vi "Create a constant from variant.vi"(5 "Terminal Sink":refnum<vi>, 6 "relative position/next to refnum":T1, 8 "error in (no error)":errorcluster, 10 "Constant Data":variant, 11 "Diagram":refnum<vi>) -> (0 "error out":errorcluster, 2 "Terminal":refnum<vi>, 3 "Const Refnum":refnum<vi>)   [LabVIEW 2018, in "Scripting Tools.lvlib"]
doc: "Create a constant on the block diagram with name and type of <b>Constant Data</b>."
uses:
  Scripting Tools.lvlib
  <vilib>/Utility/miscctls.llb/LVPointTypeDef.ctl
  <vilib>/Utility/VariantDataType/VariantType.lvlib
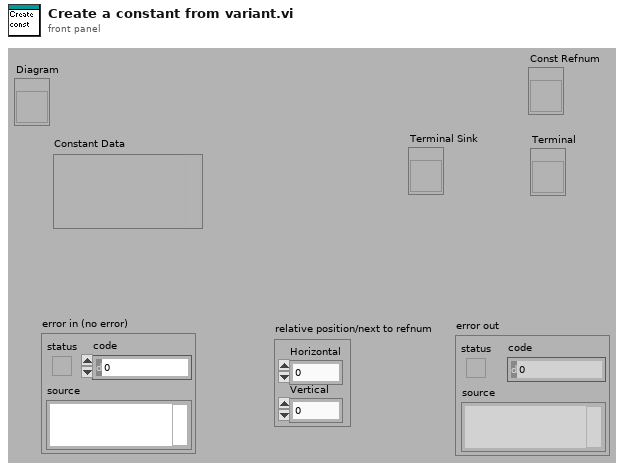
[diagram p1: front panel]
types:
  T1 = typedef "LVPointTypeDef.ctl" = cluster{"Horizontal":i16, "Vertical":i16}
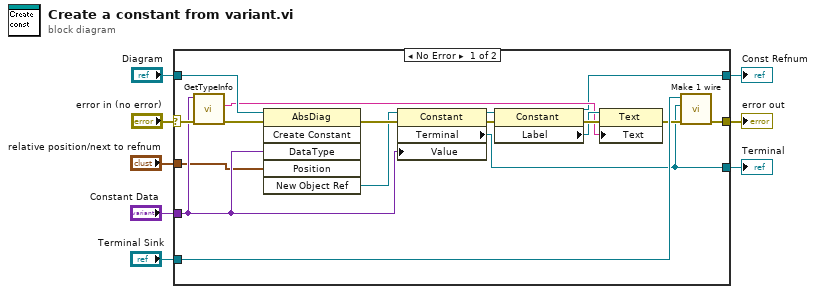
[diagram p0: block diagram]
diagram:
  n1 = case shown="No Error" "error in (no error)" {
    selector: "error in (no error)" -> [w17 w26]
    tunnel: [w25 w26] -> w7
    tunnel: "Constant Data" -> [w15 _]
    tunnel: "relative position/next to refnum" -> [w11 _]
    tunnel: "Terminal Sink" -> [w24 _]
    tunnel: "Diagram" -> [w23 _]
    tunnel: [w9 _] -> w2
    tunnel: [w12 _] -> w1
    frame No Error {
      n2 = call <vilib>:"GetTypeInfo.vi"("error in (no error)"=w17, "Variant"=w15) -> ("error out"=w16:errorcluster, "Name"=w14:string)  [unwired: 8 out]
      n3 = invoke class="AbsDiag" method="Create Constant"(reference=w23, error in=w16, "DataType"=w15, "Position"=w11) -> (error out=w22:errorcluster, "New Object Ref"=w21:refnum<vi>)  [unwired: 2 in, 4 out]
      n4 = property class="Constant"(reference=w21, error in=w22, "Value"=w15) -> (reference out=w20:refnum<vi>, error out=w10:errorcluster, "Terminal"=w9:refnum<vi>)
      n5 = property class="Constant"(reference=w20, error in=w10) -> (reference out=w12:refnum<vi>, error out=w19:errorcluster, "Label"=w18:refnum<vi>)
      n6 = property class="Text"(reference=w18, error in=w19, "Text"=w14) -> (error out=w13:errorcluster)  [unwired: 1 out]
      n7 = call "Make 1 wire.vi"("error in"=w13, "Wire Terminal 2"=w9, "Wire Terminal 1"=w24) -> ("error out"=w25:errorcluster)  [unwired: 8 out]
    }
    frame Error {
    }
  }
  "error out" <- w7
  "Const Refnum" <- w1
  "Terminal" <- w2
